vi "Request Data (unix ns).vi"(10 "Data Request":T3, 11 "Historian Module in":refnum<class "Historian Module.lvclass">) -> (2 "History Data":T1, 3 "Historian Module out":refnum<class "Historian Module.lvclass">)   [LabVIEW 2020, in "VolatusHistorian.lvlib" / "Historian Module.lvclass"]
uses:
  Historian Module.lvclass
  Data Request.ctl
  History Data (unix ns).ctl
  Channel History (unix ns).ctl
  Historian Module.lvclass/Historian Module.ctl
  Group History (unix ns).vi
  Time Filter Data (unix ns).vi
  lv-vecto/Vecto/Double Timestamp to Unix ns (Array).vi
  lv-vecto/Vecto/Double to Relative ns (Array).vi
  Group Buffer DBL/Data.vi
  VolatusHistorian.lvlib
  Time Format.ctl
panel:
  out "Unknown Channels":string[](array[string])
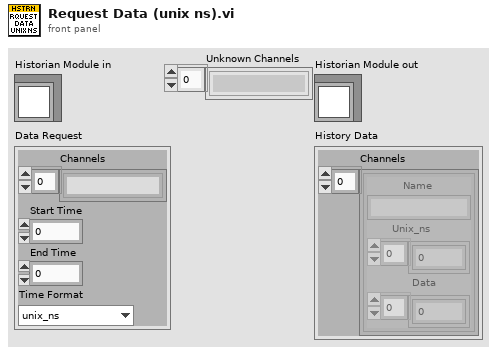
[diagram p1: front panel]
types:
  T1 = typedef "VolatusHistorian.lvlib/History Data (unix ns).ctl" = cluster{"Channels":T2[]}
  T2 = typedef "VolatusHistorian.lvlib/Channel History (unix ns).ctl" = cluster{"Name":string, "Unix_ns":i64[], "Data":dbl[]}
  T3 = typedef "VolatusHistorian.lvlib/Data Request.ctl" = cluster{"Channels":string[], "Start Time":dbl, "End Time":dbl, "Time Format":T4}
  T4 = typedef "VolatusHistorian.lvlib/Time Format.ctl" = enum16{"unix_ns", "lv"}
  T5 = typedef "VolatusHistorian.lvlib/Historian Module.lvclass/Grouped Channels.ctl" = map{string, string[]}
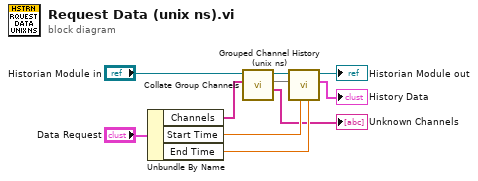
[diagram p0: block diagram]
diagram:
  n1 = Unbundle By Name("Data Request") -> ("Channels"=w8:string[], "Start Time"=w4:dbl, "End Time"=w3:dbl)
  n2 = call "Collate Group Channels.vi"("Channel Names"=w8, "Historian Module in"="Historian Module in") -> ("Unknown Channels"=→"Unknown Channels":string[], "Grouped Channels"=w5:T5, "Historian Module out"=w7:refnum<class "Historian Module.lvclass">)  [unwired: 7 in]
  n3 = call "Grouped Channel History (unix ns).vi"("End"=w3, "Start"=w4, "Grouped Channels"=w5, "Historian Module in"=w7) -> ("History Data"=→"History Data":T1, "Historian Module out"=→"Historian Module out":refnum<class "Historian Module.lvclass">)  [unwired: 6 in]
